vi "GlobalFree.vi"(4 "error in (no error)":errorcluster, 7 "hMem (NULL)":i32) -> (0 "error out":errorcluster)   [LabVIEW 2011]
uses:
  KERNEL32.DLL
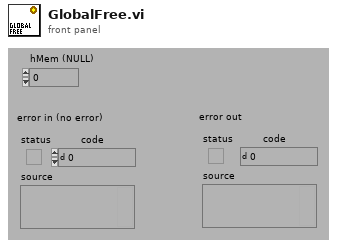
[diagram p1: front panel]
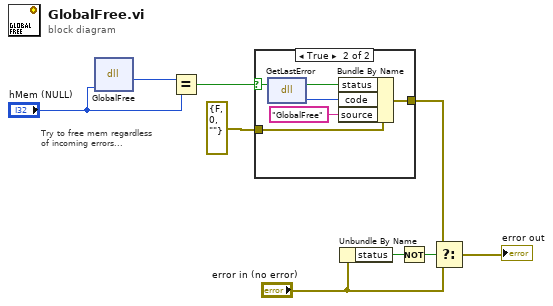
[diagram p0: block diagram]
diagram:
  # "Try to free mem regardless\nof incoming errors..."
  n1 = dll-call lib="KERNEL32.DLL" fn="GlobalFree" label="unsigned long GlobalFree(\n     unsigned long hMem);"("hMem"="hMem (NULL)") -> ("hMem"=w3:i32)  [unwired: 4 in, 2 out]
  n2 = Equal?(x=w3, y="hMem (NULL)") -> (x = y?=w1:bool)
  n3 = case shown="True" w1 {
    selector: w1 -> [_ w13]
    tunnel: [w10 w14] -> w7
    tunnel: errorcluster {"status"=FALSE, "code"=0, "source"=""} ("error out") -> [w10 w12]
    frame False {
    }
    frame True {
      n4 = dll-call lib="KERNEL32.DLL" fn="GetLastError"() -> (w11:i32)  [unwired: 3 in, 2 out]
      n5 = Bundle By Name(cluster=w12, "status"=w13, "code"=w11, "source"="GlobalFree") -> (w14:errorcluster)
    }
  }
  n6 = Unbundle By Name("error in (no error)") -> ("status"=w8:bool)
  n7 = Not(x=w8) -> (.not. x?=w5:bool)
  n8 = Select(t=w7, s=w5, f="error in (no error)") -> (s? t:f=→"error out":errorcluster)
